vi "beginKepperPassToStriker.vi"(8 "error in (no error)":errorcluster, 9 "command_interpreted":T1, 10 "Game":refnum<class "Game.lvclass">, 11 "KeeperPassToStrikerPlay in":refnum<class "KeeperPassToStrikerPlay.lvclass">) -> (0 "error out":errorcluster, 2 "beginKeeperPassToStriker":bool, 3 "KeeperPassToStrikerPlay out":refnum<class "KeeperPassToStrikerPlay.lvclass">)   [LabVIEW 2024, in "KeeperPassToStrikerPlay.lvclass"]
uses:
  KeeperPassToStrikerPlay.lvclass
  Game_class/Game.lvclass
  Referee_class/command_interpreted.ctl
  Team_class/OffensivePlay.ctl
  Game_class/Game.lvclass/Game.ctl
  Team_class/Team.lvclass/Team.ctl
  Game_class/Read OffensiveTeam.vi
  Game_class/Read Utilities.lvclass.vi
  Game_class/Read BallRef.vi
  Team_class/Read OffensivePlay.vi
  Ally_class/Ally.lvclass
  C:/Users/ROBOIME2/Documents/SSL ROBOIME/SSL_AI/Team_class/Team.lvclass
  Utilities_class/Utilities.lvclass
  Ball_class/Ball.lvclass
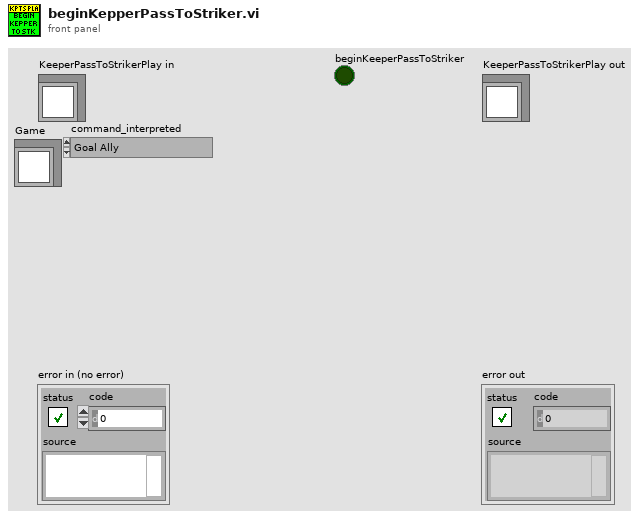
[diagram p1: front panel]
types:
  T1 = typedef "command_interpreted.ctl" = enum16{"Goal Ally", "Goal Enemy", "Ball Placement Enemy", "Ball Placement Ally", "Normal Half Time", "Extra Time  Break", "Extra Half Time", "None", "Post Game", "PKA Normal Start", "Prepare Kickoff Ally", "PKE Normal Start", "Prepare Kickoff Enemy", "Force Start", "Halt", "Timeout", "Prepare Penalty Ally", "Prepare Penalty Enemy", "PPA NormalStart", "PPE Normal Start", "Indirect Free Ally", "Direct Free Enemy", "Direct Free Ally", "Indirect Free Enemy", "Stop"}
  T2 = typedef "OffensivePlay.ctl" = enum16{"5RobotsPassGamePlay", "5PreparePassGame", "5RobotsKeeperGame", "KeeperPassToStriker", "5RobotsNormalGamePlay", "PrepareKeeperPass", "ACBPass", "ABCPass", "PrepareTriplePass", "TableWithStriker", "TableWith2ndStrikerPlay", "PrepareDoublePass", "PrepareRollToPass", "SimplePass", "PreparePass", "PassToStriker", "BallOutOfField", "PassTo2ndStriker", "StopOffensive", "Prepare Penalty Enemy", "EnemyPossessionAtEnemyField", "EnemyPossesionAtOurField", "TestPlay", "PreparePenaltyAlly", "KickPenaltyAlly", "PrepareKickoffAlly", "PrepareKickoffEnemy", "IndirectEnemy", "DirectEnemy", "PreparePassInGame1", "NormalGame", "DirectKick", "Pass", "Halt", "Timeout", "PassPlay", "PenaltyEnemy"}
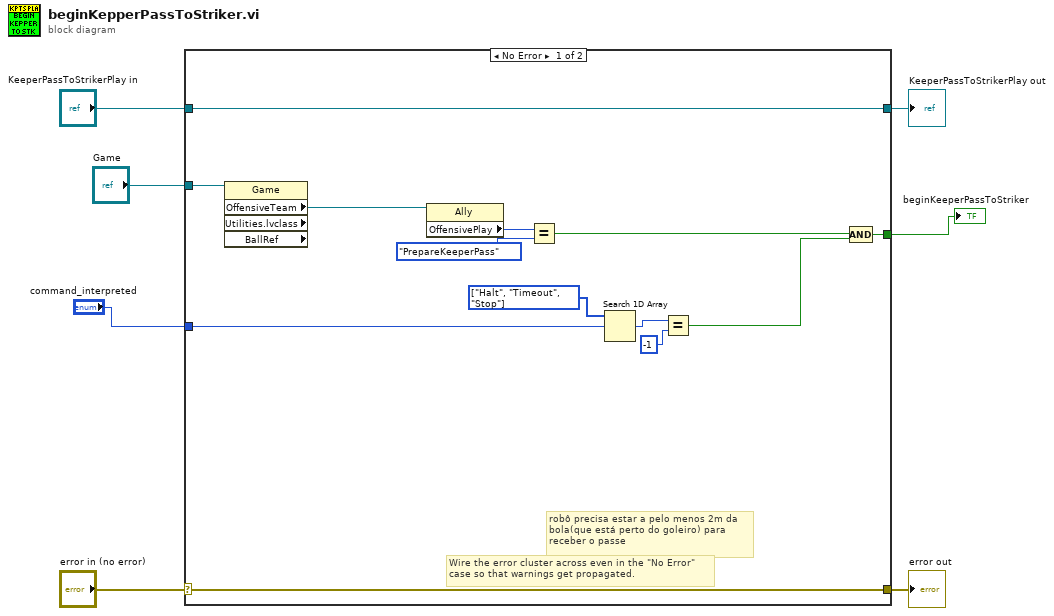
[diagram p0: block diagram]
diagram:
  n1 = case shown="No Error" "error in (no error)" {
    selector: "error in (no error)" -> [w19 w22]
    tunnel: [w19 w22] -> w6
    tunnel: [w20 w21] -> w4
    tunnel: "KeeperPassToStrikerPlay in" -> [w20 w21]
    tunnel: "Game" -> [w18 _]
    tunnel: [w14 _] -> w2
    tunnel: "command_interpreted" -> [w10 _]
    frame No Error {
      w12 = T1[] [enum."Halt", enum."Timeout", enum."Stop"] items=["Goal Ally", "Goal Enemy", "Ball Placement Enemy", "Ball Placement Ally", "Normal Half Time", "Extra Time  Break", "Extra Half Time", "None", "Post Game", "PKA Normal Start", "Prepare Kickoff Ally", "PKE Normal Start", "Prepare Kickoff Enemy", "Force Start", "Halt", "Timeout", "Prepare Penalty Ally", "Prepare Penalty Enemy", "PPA NormalStart", "PPE Normal Start", "Indirect Free Ally", "Direct Free Enemy", "Direct Free Ally", "Indirect Free Enemy", "Stop"] ("Array")
      # "robô precisa estar a pelo menos 2m da\nbola(que está perto do goleiro) para \nreceber o passe"
      # "Wire the error cluster across even in the \"No Error\"\ncase so that warnings get propagated."
      n2 = property class="Game" props=["OffensiveTeam", "Utilities.lvclass", "BallRef"](reference=w18) -> ("OffensiveTeam"=w8:refnum<class "Ally.lvclass">)  [unwired: 1 in, 4 out]
      n3 = property class="Ally"(reference=w8) -> ("OffensivePlay"=w17:T2)  [unwired: 1 in, 2 out]
      n4 = Equal?(x=w17, y=OffensivePlay."PrepareKeeperPass") -> (x = y?=w15:bool)
      n5 = Search 1D Array(1D array=w12, element=w10) -> (index of element=w13:i32)  [unwired: 1 in]
      n6 = Equal?(x=w13, y=-1) -> (x = y?=w9:bool)
      n7 = Compound Arithmetic op=AND(w15, w9) -> (w14:bool)
    }
    frame Error {
    }
  }
  "error out" <- w6
  "KeeperPassToStrikerPlay out" <- w4
  "beginKeeperPassToStriker" <- w2
